vi "PI-Connect to PIFOC.vi"(4 "error in (no error)":errorcluster) -> (0 "error out":errorcluster, 2 "PIFOC Position ACT":dbl, 3 "No Errors":bool)   [LabVIEW 2020]
uses:
  _Controls/PIFOC Settings.ctl
  _Globals/PIFOC Settings.vi
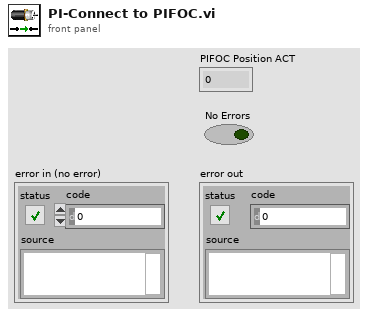
[diagram p1: front panel]
types:
  T1 = typedef "PIFOC Settings.ctl" = cluster{"System number":i32, "Commanded axes":string[], "Controller error":bool, "Error":errorcluster}
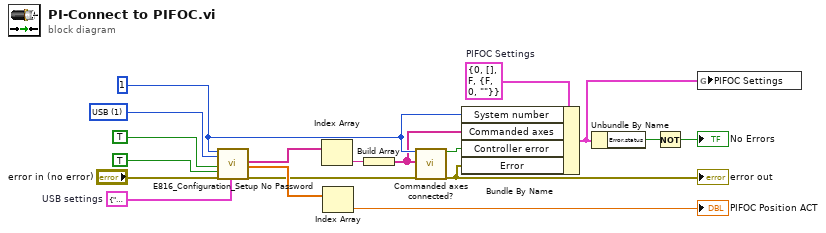
[diagram p0: block diagram]
diagram:
  w2 = T1 {"System number"=0, "Commanded axes"=[], "Controller error"=FALSE, "Error"={"status"=FALSE, "code"=0, "source"=""}}  # PIFOC Settings
  w12 = cluster{"S/N":string, "USB Search?":bool} {"S/N"="110020284", "USB Search?"=TRUE}  # USB settings
  w10 = u16 1 items=["RS232", "USB"] ("Interface")
  w5 = 1 ("System no.")
  n1 = call "E816_Configuration_Setup No Password.vi"("System no."=w5, "Interface"=w10, "All axes?"=TRUE, "Change servo \nstatus to ON?"=TRUE ("Use dialog to define\nconnected stages?"), "error in"="error in (no error)", "USB settings"=w12) -> ("Conn. Axes"=w9:string[], "Position"=w8:dbl[], "error out"=w6:errorcluster)  [unwired: 9 in, 2 out]
  n2 = Index Array(array=w9) -> (element=w7:string)  [unwired: 1 in]
  n3 = Index Array(array=w8) -> (element=→"PIFOC Position ACT":dbl)  [unwired: 1 in]
  n4 = Build Array(w7) -> (w4:string[])
  n5 = call "Commanded axes connected?.vi"("System no."=w5, "Commanded axes"=w4, "error in"=w6) -> ("Controller error"=w3:bool, "error out"=w15:errorcluster)  [unwired: 15 in]
  "error out" <- w15
  n6 = Bundle By Name(cluster=w2, "System number"=w5, "Commanded axes"=w4, "Controller error"=w3, "Error"=w15) -> (w1:T1)
  n7 = Unbundle By Name(w1) -> ("Error.status"=w13:bool)
  n8 = Not(x=w13) -> (.not. x?=→"No Errors":bool)
  n9 = global write "PIFOC Settings.vi" "PIFOC Settings"(w1) -> ()
